vi "Valco_Valve_Position.vi"(4 "Channel Name":string, 5 "Valve Number":i32(slide)=1 min=0 max=9 step=1 scale=0.0..9.0, 6 "Port Name":string, 7 "Requested Posn.":T1 items=["", "Zero Air", "Calib 1", "Calib 2", "Measure"]) -> (0 "Error Message":string, 3 "Achieved Posn.":T1 items=["", "Zero Air", "Calib 1", "Calib 2", "Measure"])   [LabVIEW 2010]
uses:
  ADAM Client/Sub VIs/ADAM Controls/Valco_valve_ph.ctl
panel:
  out "Where Next?":string
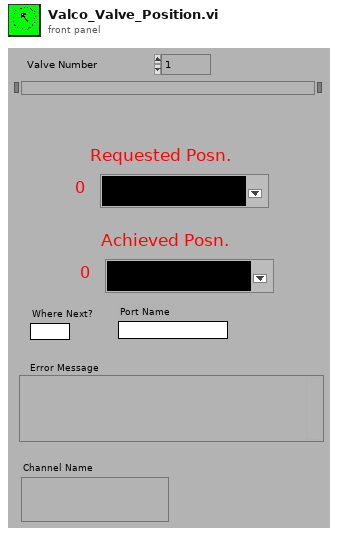
[diagram p1: front panel]
types:
  T1 = typedef "Valco_valve_ph.ctl" = u16
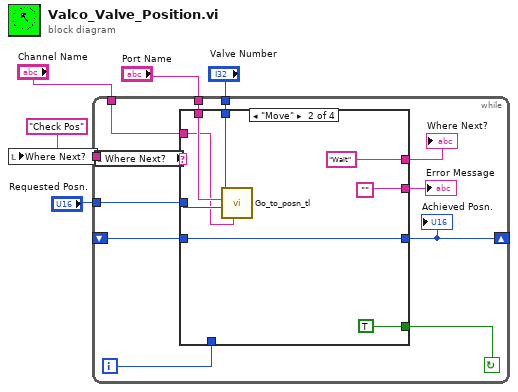
[diagram p0: block diagram]
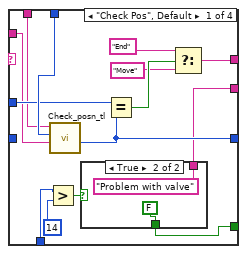
[diagram p2: hidden frame]
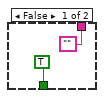
[diagram p3: hidden frame]
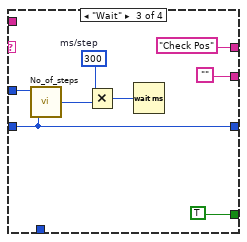
[diagram p4: hidden frame]
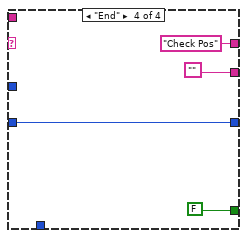
[diagram p5: hidden frame]
diagram:
  w3 = "Check Pos"
  n1 = local write "Where Next?"(w3) -> ()
  n2 = while {
    tunnel: "Channel Name" -> [w7]
    tunnel: "Port Name" -> [w8]
    tunnel: w3 -> [_]
    tunnel: "Requested Posn." -> [w13]
    shift-left: _ -> [w15]
    shift-right: [w14] -> _
    tunnel: "Valve Number" -> [w16]
    i -> [w9]
    stop <- w12 continue-if-true
    n3 = local read "Where Next?"() -> (w11:string)
    n4 = case shown="\"Move\"" w11 {
      tunnel: w16 -> [w30 w41 _ _]
      tunnel: [w28 w42 w47 w52] -> w14
      tunnel: w15 -> [_ w42 w47 w52]
      tunnel: [w27 "Wait" "Check Pos" "Check Pos"] -> w10
      tunnel: w13 -> [w29 w40 w48 _]
      tunnel: [w20 TRUE TRUE FALSE] -> w12
      tunnel: w9 -> [w23 _ _ _]
      tunnel: w8 -> [w17 w37 _ _]
      tunnel: w7 -> [w19 w36 _ _]
      tunnel: [w18 "" "" ""] -> w6
      frame "Check Pos", Default {
        n5 = Greater?(x=w23, y=14) -> (0:w21:bool)
        n6 = call "Check_posn_tl.vi"("Channel Name"=w19, "Valve Number"=w30, "Port Name"=w17) -> ("Position"=w28:i32)  [unwired: 1 in, 4 out]
        n7 = case shown="True" w21 {
          tunnel: [TRUE FALSE] -> w20
          tunnel: ["" "Problem with valve"] -> w18
          frame False {
          }
          frame True {
          }
        }
        n8 = Equal?(x=w29, y=w28) -> (x = y?=w26:bool)
        n9 = Select(t="End", s=w26, f="Move") -> (s? t:f=w27:string)
      }
      frame "Move" {
        n10 = call "Go_to_posn_tl.vi"("Channel Name"=w36, "Position"=w40, "Port Name"=w37, "Valve Number"=w41) -> ()  [unwired: 1 in, 2 out]
      }
      frame "Wait" {
        w45 = 300  # ms/step
        n11 = call "No_of_steps.vi"("Current position"=w47, "Desired position"=w48) -> ("No of steps"=w46:i32)
        n12 = Multiply(x=w45, y=w46) -> (x*y=w44:i32)
        n13 = Wait (ms)(milliseconds to wait=w44) -> ()  [unwired: 1 out]
      }
      frame "End" {
      }
    }
    "Achieved Posn." <- w14
    "Where Next?" <- w10
    "Error Message" <- w6
  }
